vi "BuildSol.vi"() -> ()   [LabVIEW 2016]
panel:
  in  "Previous Button":bool
  in  "WindowsMediaPlayer":refnum<k7>(container)
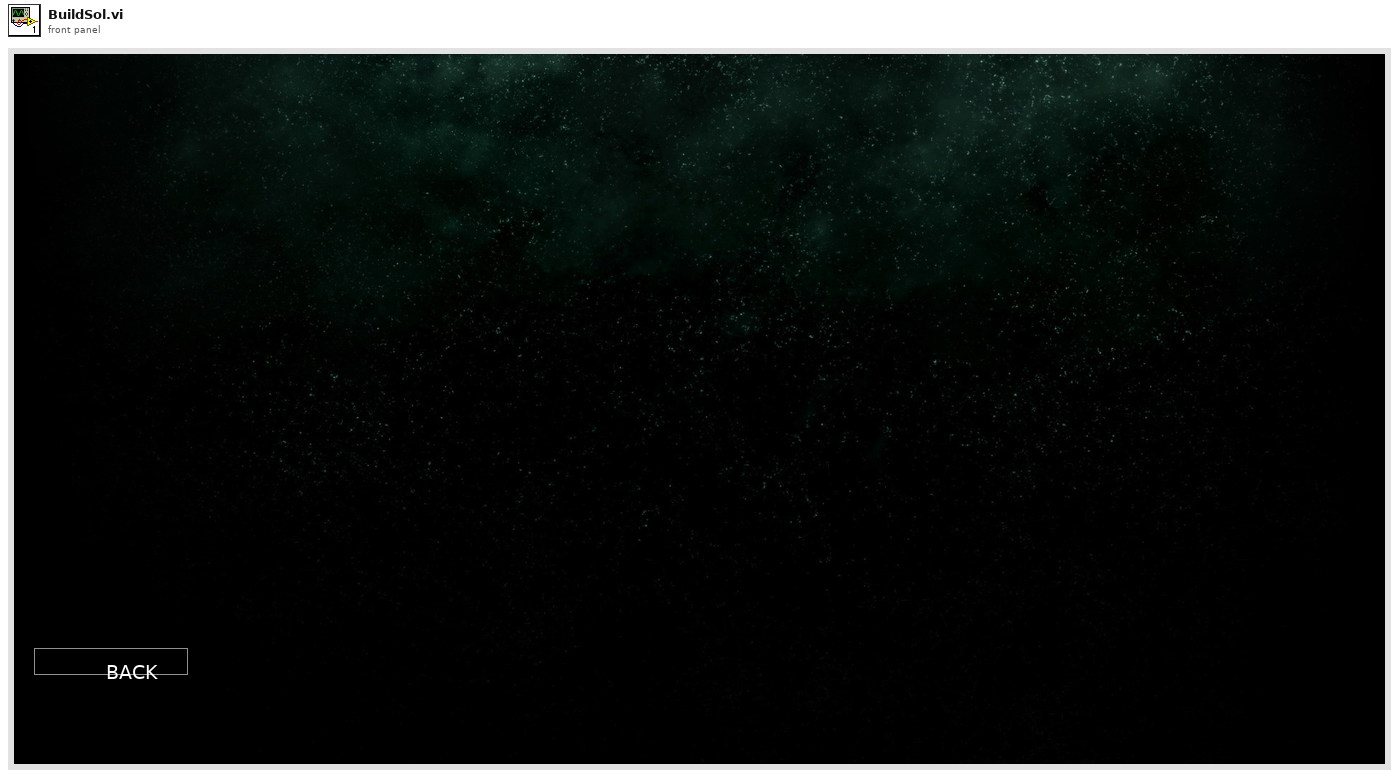
[diagram p1: front panel]
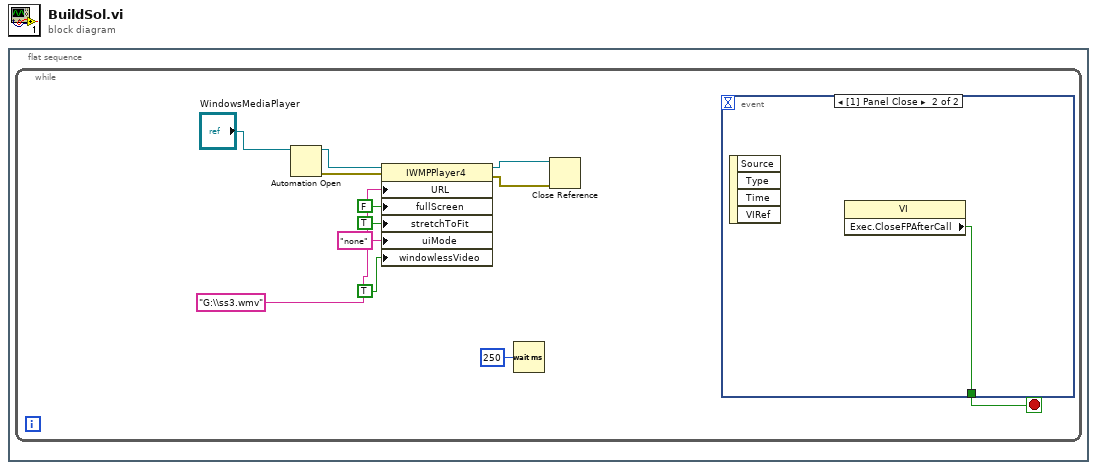
[diagram p0: block diagram]
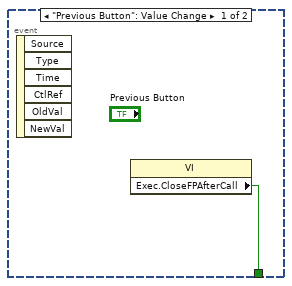
[diagram p2: hidden frame]
diagram:
  n1 = flat-sequence {
    frame #0 {
      n2 = while {
        stop <- w12 stop-if-true
        n3 = Automation Open(Automation Refnum="WindowsMediaPlayer") -> (Automation Refnum=w11:refnum<k7>, error out=w10:errorcluster)  [unwired: 3 in]
        n4 = property class="IWMPPlayer4"(reference=w11, error in=w10, "URL"="G:\\ss3.wmv", "fullScreen"=FALSE, "stretchToFit"=TRUE, "uiMode"="none", "windowlessVideo"=TRUE) -> (reference out=w9:refnum<k7>, error out=w8:errorcluster)
        n5 = Wait (ms)(milliseconds to wait=u32 250) -> ()  [unwired: 1 out]
        n6 = Close Reference(reference=w9, error in (no error)=w8) -> ()  [unwired: 1 out]
        n7 = event shown="[1] Panel Close" {
          selector: _ -> [_ _]
          dyn-events: _ -> [_ _]
          timeout: _ -> [_ _]
          tunnel: [w13 w14] -> w12
          event "Previous Button": Value Change {
            n8 = event-data() -> ()  [unwired: 1 in, 6 out]
            n9 = property class="VI"() -> ("Exec.CloseFPAfterCall"=w13:bool)  [unwired: 2 in, 2 out]
          }
          event Panel Close {
            n10 = event-data() -> ()  [unwired: 1 in, 4 out]
            n11 = property class="VI"() -> ("Exec.CloseFPAfterCall"=w14:bool)  [unwired: 2 in, 2 out]
          }
        }
      }
    }
  }
